vi "GetOwningNode.vi"(6 "error in":errorcluster, 9 "Terminal in":refnum<class "Terminal.lvclass">) -> (0 "error out":errorcluster, 3 "Terminal out":refnum<class "Terminal.lvclass">, 4 "node UID":i32)   [LabVIEW 2014, in "Raspberry Pi Compatible Compiler for LabVIEW.lvlib" / "Terminal.lvclass"]
uses:
  Terminal.lvclass
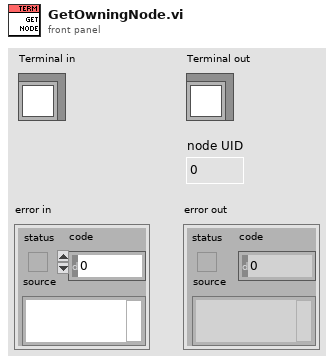
[diagram p1: front panel]
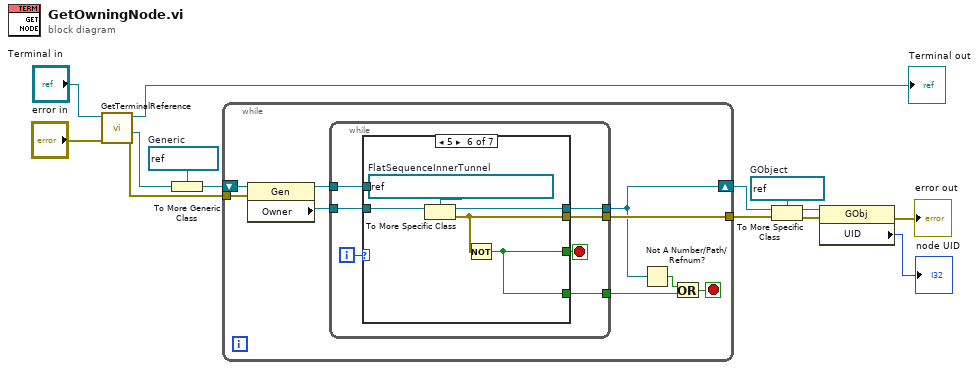
[diagram p0: block diagram]
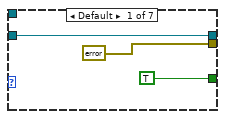
[diagram p2: hidden frame]
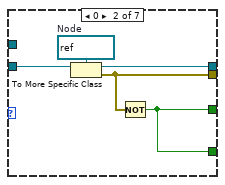
[diagram p3: hidden frame]
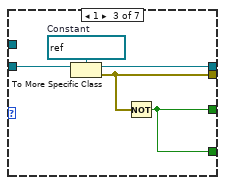
[diagram p4: hidden frame]
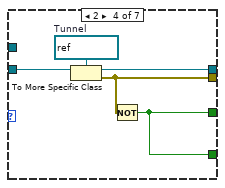
[diagram p5: hidden frame]
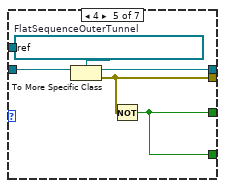
[diagram p6: hidden frame]
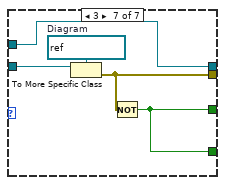
[diagram p7: hidden frame]
diagram:
  w5 = refnum<vi> refnum  # GObject
  w10 = refnum<vi> refnum  # Generic
  n1 = call "GetTerminalReference.vi"("error in"="error in", "Terminal in"="Terminal in") -> ("error out"=w11:errorcluster, "reference"=w8:refnum<vi>, "Terminal out"=→"Terminal out":refnum<class "Terminal.lvclass">)  [unwired: 7 in]
  n2 = To More Generic Class(target class=w10, reference=w8) -> (generic class reference=w9:refnum<vi>)
  n3 = while {
    tunnel: w11 -> [w22]
    shift-right: [w17] -> w3
    shift-left: w9 -> [w23]
    tunnel: [w20] -> w4
    stop <- w18 stop-if-true
    n4 = property class="Gen"(reference=w23, error in=w22) -> (reference out=w15:refnum<vi>, "Owner"=w21:refnum<vi>)  [unwired: 1 out]
    n5 = while {
      tunnel: w21 -> [w29]
      tunnel: [w27] -> w17
      tunnel: [w26] -> w20
      tunnel: [w25] -> w19
      tunnel: w15 -> [w24]
      i -> [w30]
      stop <- w28 stop-if-true
      n6 = case shown="5" w30 {
        tunnel: w29 -> [w31 w37 w42 w47 w52 w57 w62]
        tunnel: [errorcluster {"status"=TRUE, "code"=666, "source"="Term Owner"} ("error out") w36 w41 w45 w50 w55 w61] -> w26
        tunnel: [TRUE w34 w39 w44 w49 w54 w60] -> w28
        tunnel: [w31 w35 w40 w46 w51 w56 w59] -> w27
        tunnel: [_ w34 w39 w44 w49 w54 w60] -> w25
        tunnel: w24 -> [_ _ _ _ _ _ w59]
        frame Default {
        }
        frame 0 {
          w38 = refnum<vi> refnum  # Node
          n7 = To More Specific Class(target class=w38, reference=w37) -> (specific class reference=w35:refnum<vi>, error out=w36:errorcluster)  [unwired: 1 in]
          n8 = Not(x=w36) -> (.not. x?=w34:bool)
        }
        frame 1 {
          w43 = refnum<vi> refnum  # Constant
          n9 = To More Specific Class(target class=w43, reference=w42) -> (specific class reference=w40:refnum<vi>, error out=w41:errorcluster)  [unwired: 1 in]
          n10 = Not(x=w41) -> (.not. x?=w39:bool)
        }
        frame 2 {
          w48 = refnum<vi> refnum  # Tunnel
          n11 = To More Specific Class(target class=w48, reference=w47) -> (specific class reference=w46:refnum<vi>, error out=w45:errorcluster)  [unwired: 1 in]
          n12 = Not(x=w45) -> (.not. x?=w44:bool)
        }
        frame 4 {
          w53 = refnum<vi> refnum  # FlatSequenceOuterTunnel
          n13 = To More Specific Class(target class=w53, reference=w52) -> (specific class reference=w51:refnum<vi>, error out=w50:errorcluster)  [unwired: 1 in]
          n14 = Not(x=w50) -> (.not. x?=w49:bool)
        }
        frame 5 {
          w58 = refnum<vi> refnum  # FlatSequenceInnerTunnel
          n15 = To More Specific Class(target class=w58, reference=w57) -> (specific class reference=w56:refnum<vi>, error out=w55:errorcluster)  [unwired: 1 in]
          n16 = Not(x=w55) -> (.not. x?=w54:bool)
        }
        frame 3 {
          w63 = refnum<vi> refnum  # Diagram
          n17 = To More Specific Class(target class=w63, reference=w62) -> (error out=w61:errorcluster)  [unwired: 1 in, 1 out]
          n18 = Not(x=w61) -> (.not. x?=w60:bool)
        }
      }
    }
    n19 = Not A Number/Path/Refnum?(number/path/refnum=w17) -> (NaN/Path/Refnum?=w16:bool)
    n20 = Or(x=w16, y=w19) -> (x .or. y?=w18:bool)
  }
  n21 = To More Specific Class(target class=w5, reference=w3, error in=w4) -> (specific class reference=w6:refnum<vi>, error out=w7:errorcluster)
  n22 = property class="GObj"(reference=w6, error in=w7) -> (error out=→"error out":errorcluster, "UID"=→"node UID":i32)  [unwired: 1 out]
